vi "Dashboard Main.vi"() -> ()   [LabVIEW 2014]
uses:
  Typedefs/StackerStates.ctl
  Typedefs/Arm States.ctl
  Typedefs/ClawStates.ctl
  <vilib>/event_ctls.llb/eventvkey.ctl
  <vilib>/Rock Robotics/WPI/Dashboard/WPI_DashboardLogging Global.vi
  <vilib>/Rock Robotics/Network Tables/SD Read Boolean.vi
  <vilib>/Rock Robotics/Network Tables/SD Read Number.vi
  <vilib>/Rock Robotics/Network Tables/SD Read String Array.vi
  <vilib>/Utility/config.llb/Write Key (String).vi
  <vilib>/Utility/config.llb/Write Key (I32).vi
  <vilib>/Utility/config.llb/NI_LVConfig.lvlib
panel:
  in  "TCP":refnum<k5>
  in  "Rec Mode":enum32{"Stop", "Record", "Playback"}(radio)
  in  "Vision":u16(ring) items=["Camera Off", "USB Camera SW", "USB Camera HW", "IP Camera"]
  out "Camera IP":string
  out "Image Message":string="Timeout in Camera Communications"
  in  "Dashboard Tab":T1(tab)
  in  "Camera Settings":T2={"Frame Rate"=30, "Compression"=30, "Size"=1} {"Frame Rate" scale=1.0..30.0; "Size" items=["640x480", "320x240", "160x120"]}
  out "MotorChart R":cluster{"Numeric":dbl, "Numeric":dbl}(graph)
  out "MotorChart L":T3(graph)
  out "MotorSliders R":cluster{"MotorSlide1":dbl, "MotorSlide2":dbl} {"MotorSlide2" scale=-1.0..1.0 scale format="%#_2e"; "MotorSlide1" scale=-1.0..1.0 scale format="%#_2e"}
  out "MotorSliders L":T4 {"MotorSlide4 2" scale=0.0..14.0 scale format="%#_2e"; "MotorSlide2" scale=-1.0..1.0 scale format="%#_2e"; "MotorSlide1" scale=-1.0..1.0 scale format="%#_2e"}
  out "Gyro":dbl(knob) scale=0.0..360.0
  out "JS1 Z":dbl(slide) scale=-1.0..1.0 scale format="%#_2e"
  out "JS1 Graph":cluster{"X":dbl, "Y":dbl}[](graph)
  out "JS1 Buttons":T5
  out "JS2 Z":dbl(slide) scale=-1.0..1.0 scale format="%#_2e"
  out "JS2 Graph":cluster{"X":dbl, "Y":dbl}[](graph)
  out "JS2 Buttons":T5
  out "Mode":T6(ring)=enum."Auto Disabled"
  in  "DB Camera Config":bool
  out "fps":dbl format="%#.1g"
  out "Mbps":dbl format="%#.1g"
  out "Mbps 2":bool
  in  "DB/String 9":string
  in  "DB/String 8":string
  in  "DB/String 7":string
  in  "DB/String 6":string
  in  "DB/String 5":string
  in  "DB/String 4":string
  in  "DB/String 3":string
  in  "DB/String 2":string
  in  "DB/String 1":string
  in  "DB/String 0":string
  in  "DB/Slider 0":dbl(slide) scale=0.0..5.0
  in  "DB/Slider 1":dbl(slide) scale=0.0..5.0
  in  "DB/Slider 2":dbl(slide) scale=0.0..5.0
  in  "DB/Slider 3":dbl(slide) scale=0.0..5.0
  out "DB/LED 3":bool
  out "DB/LED 2":bool
  out "DB/LED 1":bool
  out "DB/LED 0":bool
  in  "DB/Button 3":bool
  in  "DB/Button 2":bool
  in  "DB/Button 1":bool
  in  "DB/Button 0":bool caption="New Name"
  out "Claw On":bool
  out "Intake On":bool
  out "Right Throttle":dbl
  out "Comp Bot":bool
  out "Intake Sensor Enabled":bool
  out "Number of Totes":u8
  out "Compressor On":bool
  out "Intake Sees Tote":bool
  out "Stacker Sees Tote":bool
  out "Tusks Up":bool
  out "Stacker On":bool
  out "Compressor Enabled":bool
  out "Stacker State to Index":T7
  out "Arm State":T8
  out "Claw State":T9
  out "Auto Mode":string
  out "Left Throttle":dbl
  out "Claw Sees Can":bool
  out "Stack Clamp Locked?":bool
  in  "Test Slider":dbl(slide) scale=0.0..100.0 scale format="%#_3g"
  in  "On/Off":bool caption="Solenoid"
  in  "Test Name":u16(ring) items=["Select the test to run...", "Example Test", "-------------------------------", "List of tests is built in robot code.", "Replace with your own automated tests."]
  in  "Test Tree":string(tree)
  in  "Motor":cluster{"Value":dbl, "Enable":bool} {"Value" scale=-1.0..1.0 scale format="%#_3g"}
  out "Progress":T10 {"Test Progress" scale=0.0..100.0}
  in  "Rev/Fwd":cluster{"Forward":bool, "Reverse":bool}
  in  "Test Ring":u16(ring) items=["Monochrome", "Color"]
  in  "Listbox":i32(listbox)
  out "Tree":string(tree)
  out "Camera Image":T11(plugin-control)
  out "Boolean":bool
  # "Left"
  # "Front"
  # "Right"
  # "Battery"
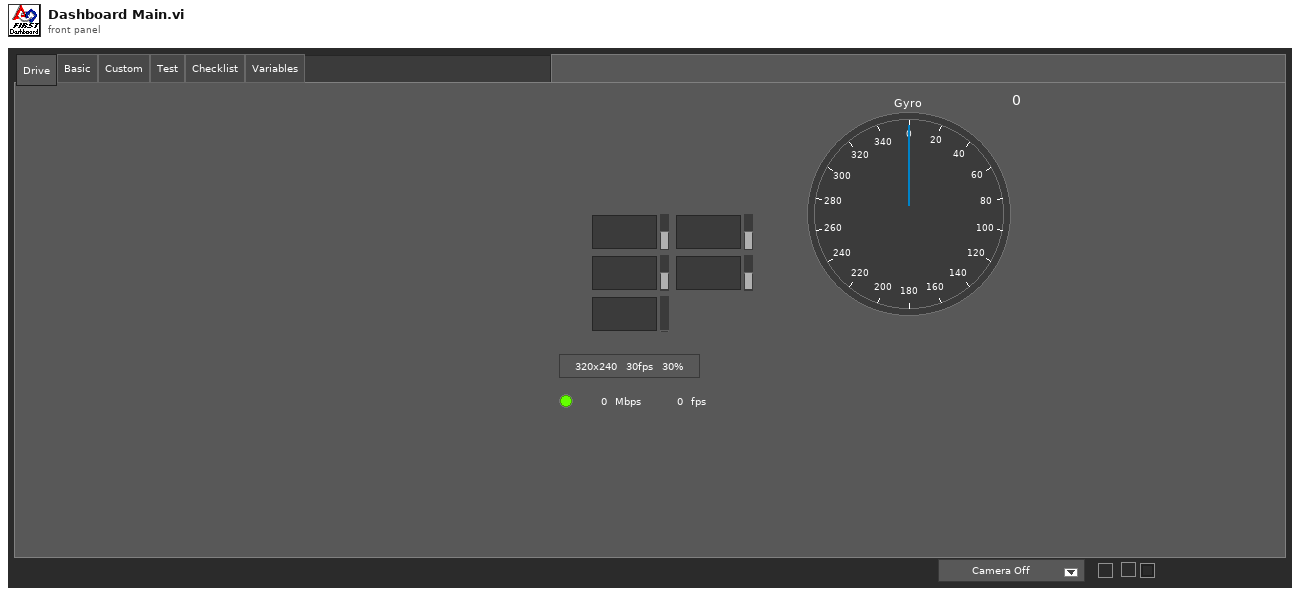
[diagram p1: front panel]
types:
  T1 = enum32{"Drive", "Basic", "Custom", "Test", "Checklist", "Variables"}
  T2 = cluster{"Frame Rate":i32, "Compression":i32, "Size":u16}
  T3 = cluster{"Numeric":dbl, "Numeric":dbl, "Battery V":dbl}
  T4 = cluster{"MotorSlide1":dbl, "MotorSlide2":dbl, "MotorSlide4 2":dbl}
  T5 = cluster{bool, bool, bool, bool, bool, bool, bool, bool, bool, bool, bool, bool}
  T6 = enum8{"Tele-Op Disabled", "Tele-Op Enabled", "Auto Disabled", "Auto Enabled", "Test Disabled", "Test Enabled", "Disconnected", "No Code", "E-Stop"}
  T7 = typedef "StackerStates.ctl" = enum16{"Manual ", "Hold", "Hold5", "Hold6", "GetTote", "DropStack", "Hover", "Hover5", "Wait for Up", "DecideHold", "DownTimerPeriod", "Prep Intake for Drop", "Check Arm before 5", "Make Arm ready for 5", "Check Arm before 6", "Make Arm ready for 6", "Delay for 5", "Delay for 6"}
  T8 = typedef "Arm States.ctl" = enum16{"Arm Manual ", "Ground", "Step", "1 Tote", "2 Tote", "3 Tote", "4 Tote", "5 Tote", "6 Tote", "Flip Can Arm", "Grab Can in auto"}
  T9 = typedef "ClawStates.ctl" = enum16{"Claw Manual ", "Claw Open", "Claw Closed", "Claw Slight Open", "Flip Can"}
  T10 = cluster{"Test Progress":u8, "Test Progress Text":string}
  T11 = typedef "IMAQ Image.ctl" = refnum<image>
  T12 = typedef "Image Type" = u32
  T13 = cluster{"Camera Image":refnum<vi>, "Dashboard Tab":refnum<vi>, "Boolean":refnum<vi>, "Vision":refnum<vi>, "Rec Mode":refnum<vi>, "Test Slider":refnum<vi>, "On/Off ":refnum<vi>, "Test Ring":refnum<vi>, "Rev/Fwd":refnum<vi>, "Test Name":refnum<vi>, "Motor":refnum<vi>, "Progress":refnum<vi>, "CheckList":refnum<vi>, "Tree":refnum<vi>, "Test Tree":refnum<vi>}
  T14 = cluster{"Error Strings":string, "Disable Counts":cluster{u16, u16}, "Rail Faults":cluster{u16, u16, u16}, "Robot IP":string, "DB Mode":u8, "Event Info":cluster{"Name":string, "Type":u8, "Number":u16, "Replay":u8}, "Camera Addr":string}
  T15 = cluster{"Storage":cluster{"Disk Free":u64, "RAM Block":u32, "RAM free":u32}, "CPU Utilization":cluster{"CPU % ISR":sgl, "CPU % Time Crit":sgl, "CPU % Timed Str":sgl, "CPU % High":sgl, "CPU % Above":sgl, "CPU % Normal":sgl, "CPU % Low":sgl}, "CAN":cluster{"% Bus Utilization":sgl, "Bus Off Cnt":u32, "TX_FIFO Full Cnt":u32, "Receive Error Cnt":u8, "Transmit Error Cnt":u8}, "HID":cluster{"HID Outputs":u32, "Rumble Low":u16, "Rumble High":u16}[]}
  T16 = cluster{"Status bits":cluster{"Test Mode":bool, "Autonomous":bool, "Enabled":bool, "Code Start":bool, "Brownout":bool, "Reserved 2":bool, "Reserved 3":bool, "E-Stop":bool}, "Code Trace":cluster{"Disabled":bool, "TeleOp":bool, "Auto":bool, "Test":bool}, "Controller Type":enum16{"unknown", "cRIO", "roboRio"}, "Code?":enum16{"unknown", "noCode", "code"}, "Battery V":dbl}
  T17 = cluster{"Control Bits":cluster{"TestMode":bool, "Autonomous":bool, "Enabled":bool, "FMS Present":bool, bool, bool, bool, "E-Stop":bool}, "Team Station ":u8, "Countdown":sgl, "Joystick Values":cluster{"Axes":dbl[], "Buttons":bool[], "POVs":i16[]}[]}
  T18 = cluster{"Axes":dbl[], "Buttons":bool[], "POVs":i16[]}[]
  T19 = cluster{"Axes":dbl[], "Buttons":bool[], "POVs":i16[]}
  T20 = cluster{"Buttons[0]":bool, "Buttons[1]":bool, "Buttons[2]":bool, "Buttons[3]":bool, "Buttons[4]":bool, "Buttons[5]":bool, "Buttons[6]":bool, "Buttons[7]":bool, "Buttons[8]":bool, "Buttons[9]":bool, "Buttons[10]":bool, "Buttons[11]":bool}
  T21 = typedef "NI_LVConfig.lvlib/Config Data RefNum.ctl" = refnum<k1>
  T22 = cluster{"Operation":enum16{"Update", "Clear"}, "Color Box":u32}[]
  T23 = typedef "eventvkey.ctl" = enum16{"ASCII", "Enter", "Return", "Shift", "Ctrl", "Alt", "Cmd", "Opt", "Caps", "NumLock", "Clear", "Break", "Up", "Down", "Left", "Right", "Insert", "Delete", "Home", "End", "PageUp", "PageDown", "Escape", "Help", "Pause", "ScrollLock", "F1", "F2", "F3", "F4", "F5", "F6", "F7", "F8", "F9", "F10", "F11", "F12", "F13", "F14", "F15", "F16", "F17", "F18", "F19", "F20", "F21", "F22", "F23", "F24", "Play", "VolumeUp", "VolumeDown", "Mute", "Two Byte Char"}
  T24 = cluster{"Image Size":bool, "Image Type":bool, "Pixel Value":bool, "ROI Information":bool, "Zoom Factor":bool}
  T25 = enum8{"Enabled", "Disabled", "Disabled and Grayed Out"}
  T26 = cluster{"Operation":enum16{"Update", "Clear"}, "Color Box":u32}
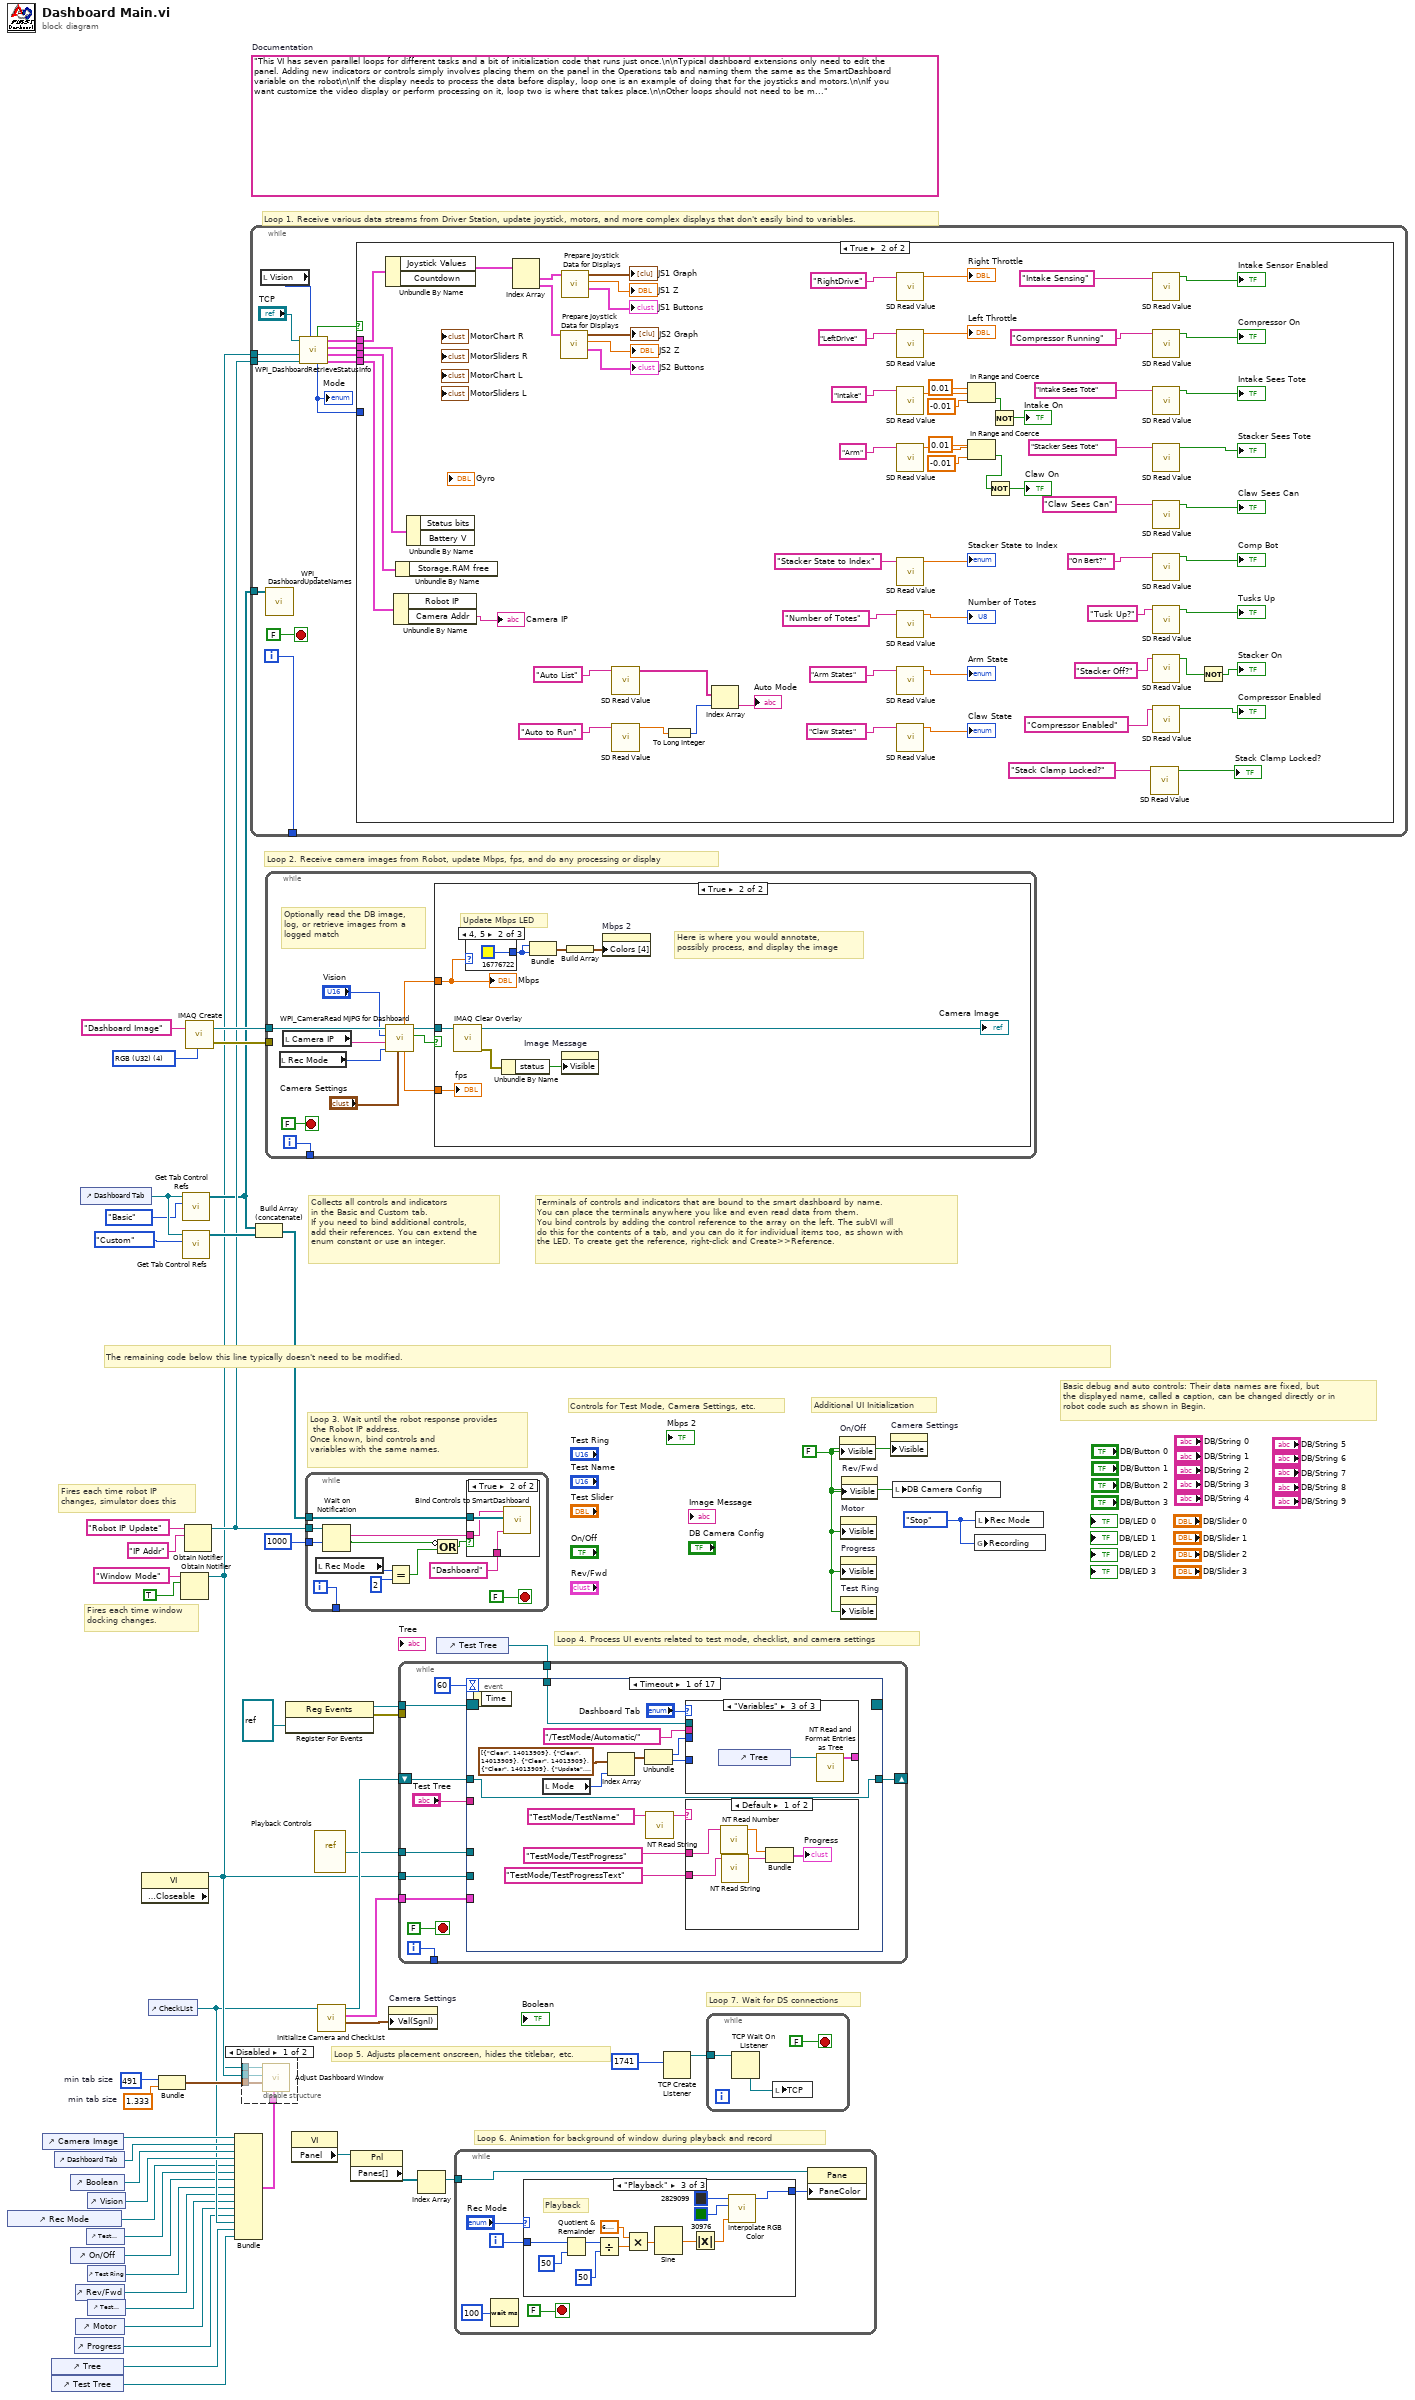
[diagram p0: block diagram]
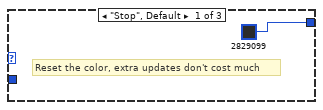
[diagram p4: hidden frame]
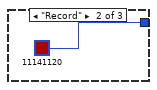
[diagram p5: hidden frame]
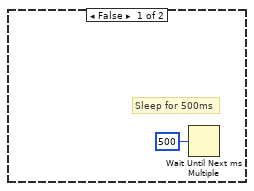
[diagram p7: hidden frame]
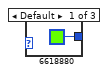
[diagram p8: hidden frame]
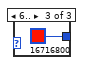
[diagram p9: hidden frame]
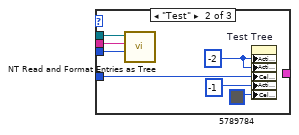
[diagram p11: hidden frame]
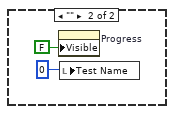
[diagram p12: hidden frame]
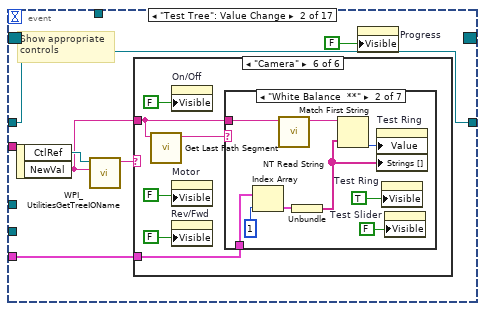
[diagram p13: hidden frame]
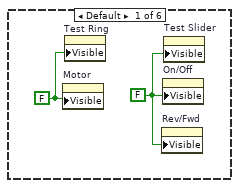
[diagram p14: hidden frame]
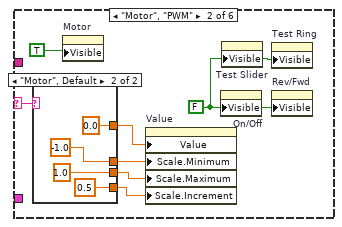
[diagram p15: hidden frame]
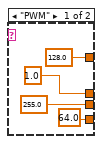
[diagram p16: hidden frame]
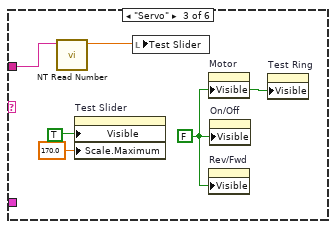
[diagram p17: hidden frame]
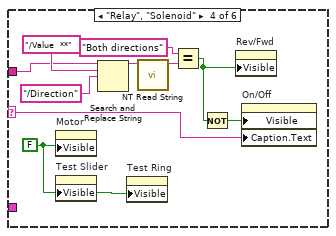
[diagram p18: hidden frame]
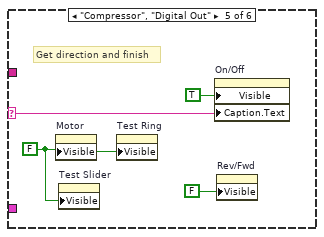
[diagram p19: hidden frame]
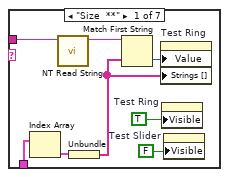
[diagram p20: hidden frame]
diagram:
  w24 = 491  # min tab size
  w23 = 1.333  # min tab size
  w32 = enum32{"Stop", "Record", "Playback"}."Stop" ("Rec Mode")
  w6 = FALSE ("Visible")
  (unwired) "This VI has seven parallel loops for different tasks and a bit of initialization code that runs just once.\n\nTypical dashboard extensions only need to edit the panel. Adding new indicators or controls simply involves placing them on the panel in the Operations tab and naming them the same as the SmartDashboard variable on the robot\n\nIf the display needs to process the data before display, loop one is an example of doing that for the joysticks and motors.\n\nIf you want customize the video display or perform processing on it, loop two is where that takes place.\n\nOther loops should not need to be modified. They are pretty standard, and document the task they perform."  # Documentation
  w52 = T12 4 items=["Grayscale (U8)", "Grayscale (I16)", "Grayscale (SGL)", "Complex (CSG)", "RGB (U32)", "HSL (U32)", "RGB (U64)"] ("Image Type")
  # "Loop 7. Wait for DS connections"
  # "Basic debug and auto controls: Their data names are fixed, but\nthe displayed name, called a caption, can be changed directly or in\nrobot code such as shown in Begin."
  # "Controls for Test Mode, Camera Settings, etc."
  # "Additional UI Initialization"
  # "Loop 6. Animation for background of window during playback and record"
  # "Fires each time robot IP\nchanges, simulator does this"
  # "Fires each time window\ndocking changes."
  # "Collects all controls and indicators\nin the Basic and Custom tab.\nIf you need to bind additional controls,\nadd their references. You can extend the\nenum constant or use an integer."
  # "The remaining code below this line typically doesn't need to be modified."
  # "Loop 4. Process UI events related to test mode, checklist, and camera settings"
  # "Terminals of controls and indicators that are bound to the smart dashboard by name.\nYou can place the terminals anywhere you like and even read data from them.\nYou bind controls by adding the control reference to the array on the left. The subVI will\ndo this for the contents of a tab, and you can do it for individual items too, as shown with\nthe LED. To create get the reference, right-click and Create>>Reference."
  # "Loop 3. Wait until the robot response provides\n the Robot IP address.\nOnce known, bind controls and\nvariables with the same names."
  # "Loop 5. Adjusts placement onscreen, hides the titlebar, etc."
  # "Loop 1. Receive various data streams from Driver Station, update joystick, motors, and more complex displays that don't easily bind to variables."
  # "Loop 2. Receive camera images from Robot, update Mbps, fps, and do any processing or display"
  n1 = control-ref of="Rec Mode"() -> (w12:refnum<vi>)
  n2 = control-ref of="Camera Image"() -> (w27:refnum<vi>)
  n3 = control-ref of="Tree"() -> (w16:refnum<vi>)
  n4 = control-ref of="Test Tree"() -> (w15:refnum<vi>)
  n5 = control-ref of="Dashboard Tab"() -> (w26:refnum<vi>)
  n6 = control-ref of="Boolean"() -> (w21:refnum<vi>)
  n7 = control-ref of="On/Off"() -> (w10:refnum<vi>)
  n8 = control-ref of="Progress"() -> (w7:refnum<vi>)
  n9 = control-ref of="Rev/Fwd"() -> (w8:refnum<vi>)
  n10 = control-ref of="Motor"() -> (w13:refnum<vi>)
  n11 = control-ref of="Dashboard Tab"() -> (w30:refnum<vi>)
  n12 = control-ref of="Test Slider"() -> (w11:refnum<vi>)
  n13 = control-ref of="Vision"() -> (w25:refnum<vi>)
  n14 = control-ref of="Test Ring"() -> (w9:refnum<vi>)
  n15 = control-ref of="Test Name"() -> (w14:refnum<vi>)
  n16 = property class="VI" props=["Front Panel.Closeable"]() -> (reference out=w31:refnum<vi>)  [unwired: 2 in, 2 out]
  n17 = control-ref of="CheckList"() -> (w17:refnum<vi>)
  n18 = Bundle("min tab size"=w24, "min tab size"=w23) -> (w22:cluster{"min tab size":i32, "min tab size":dbl})  [unwired: 1 in]
  n19 = Obtain Notifier(name (unnamed)="Window Mode", notification data type=TRUE) -> (notifier out=w3:refnum<notifier>)  [unwired: 2 in, 2 out]
  n20 = call <vilib>:"Get Tab Control Refs.vi"("Page Index"=T1."Basic" ("Dashboard Tab"), "TabControl in"=w30) -> ("ControlsOnPage"=w4:refnum<vi>[])  [unwired: 9 in]
  n21 = call <vilib>:"Get Tab Control Refs.vi"("Page Index"=T1."Custom" ("Dashboard Tab"), "TabControl in"=w30) -> ("ControlsOnPage"=w29:refnum<vi>[])  [unwired: 9 in]
  n22 = Obtain Notifier(name (unnamed)="Robot IP Update", notification data type="IP Addr" ("name (unnamed)")) -> (notifier out=w5:refnum<notifier>)  [unwired: 2 in, 2 out]
  n23 = call "IMAQ Create"("Image Name"="Dashboard Image", "Image Type"=w52) -> ("New Image"=w50:T11, "error out"=w49:errorcluster)  [unwired: 2 in, 1 out]
  n24 = Bundle("Camera Image"=w27, "Dashboard Tab"=w26, "Boolean"=w21, "Vision"=w25, "Rec Mode"=w12, "Test Slider"=w11, "On/Off"=w10, "Test Ring"=w9, "Rev/Fwd"=w8, "Test Name"=w14, "Motor"=w13, "Progress"=w7, "CheckList"=w17, "Tree"=w16, "Test Tree"=w15) -> (w18:T13)  [unwired: 1 in]
  n25 = disable-structure shown="Disabled" {
    disable-tunnel: w31 -> [w56 _]
    disable-tunnel: w22 -> [w55 _]
    disable-tunnel: w18 -> [w54 _]
    disable-tunnel: w3 -> [w53 _]
    frame Disabled {
      n26 = call "Adjust Dashboard Window.vi"("Sizing Refnums"=w54, "Size Constraints"=w55, "VI"=w56, "Notifier in"=w53) -> ()  [unwired: 8 in]
    }
    frame Enabled {
    }
  }
  n27 = while {
    tunnel: [w68] -> _
    tunnel: w5 -> [w62]
    tunnel: w4 -> [w61]
    tunnel: w3 -> [w57]
    i -> [w68]
    stop <- FALSE stop-if-true
    n28 = local read "Vision"() -> (w59:u16)
    n29 = call <vilib>:"WPI_DashboardUpdateNames.vi"("Controls on Tab"=w61) -> ()  [unwired: 11 in]
    n30 = call <vilib>:"WPI_DashboardRetrieveStatusInfo.vi"("Vision"=w59, "Binding Refnum"=w62, "Window Mode Notifier"=w57, "TCP Cnx"="TCP") -> ("Power and Errors"=w63:T14, "Robot Metrics"=w66:T15, "Status Info"=w67:T16, "Control Info"=w64:T17, "Robot Mode"=w60:T6, "Process?"=w65:bool)  [unwired: 2 in]
    "Mode" <- w60
    n31 = case shown="True" w65 {
      tunnel: w67 -> [_ w134]
      tunnel: w66 -> [_ w133]
      tunnel: w64 -> [_ w132]
      tunnel: w63 -> [_ w131]
      tunnel: w60 -> [_ _]
      frame False {
      }
      frame True {
        n32 = Unbundle By Name(w132) -> ("Joystick Values"=w130:T18)  [unwired: 1 out]
        n33 = Unbundle By Name(w131) -> ("Camera Addr"=→"Camera IP":string)  [unwired: 1 out]
        n34 = Unbundle By Name(w133) -> ()  [unwired: 1 out]
        n35 = Unbundle By Name(w134) -> ()  [unwired: 2 out]
        n36 = Index Array(array=w130) -> (element #1=w129:T19, element #2=w124:T19)  [unwired: 2 in]
        n37 = call "Prepare Joystick Data for Displays.vi"("Joystick Values"=w124) -> ("Buttons"=→"JS2 Buttons":T20, "Z Axis"=→"JS2 Z":dbl, "Cartesian Data"=→"JS2 Graph":cluster{"X axis":dbl, "X axis":dbl}[])  [unwired: 8 in]
        n38 = call "Prepare Joystick Data for Displays.vi"("Joystick Values"=w129) -> ("Buttons"=→"JS1 Buttons":T20, "Z Axis"=→"JS1 Z":dbl, "Cartesian Data"=→"JS1 Graph":cluster{"X axis":dbl, "X axis":dbl}[])  [unwired: 8 in]
        n39 = call-poly <vilib>:"SD Read Value.vi"("Name"="Auto List") -> ("String Array"=w89:string[])  [unwired: 9 in, 1 out]
        n40 = call-poly <vilib>:"SD Read Value.vi"("Name"="Auto to Run") -> ("Numeric"=w88:dbl)  [unwired: 8 in, 2 out]
        n41 = To Long Integer(number=w88) -> (32bit integer=w87:i32)
        n42 = Index Array(array=w89, index=w87) -> (element=→"Auto Mode":string)
        n43 = call-poly <vilib>:"SD Read Value.vi"("Name"="RightDrive") -> ("Numeric"=→"Right Throttle":dbl)  [unwired: 8 in, 2 out]
        n44 = call-poly <vilib>:"SD Read Value.vi"("Name"="LeftDrive") -> ("Numeric"=→"Left Throttle":dbl)  [unwired: 8 in, 2 out]
        n45 = call-poly <vilib>:"SD Read Value.vi"("Name"="Intake") -> ("Numeric"=w83:dbl)  [unwired: 8 in, 2 out]
        n46 = call-poly <vilib>:"SD Read Value.vi"("Name"="Arm") -> ("Numeric"=w78:dbl)  [unwired: 8 in, 2 out]
        n47 = call-poly <vilib>:"SD Read Value.vi"("Name"="Stacker State to Index") -> ("Numeric"=→"Stacker State to Index":dbl)  [unwired: 8 in, 2 out]
        n48 = call-poly <vilib>:"SD Read Value.vi"("Name"="Number of Totes") -> ("Numeric"=→"Number of Totes":dbl)  [unwired: 8 in, 2 out]
        n49 = call-poly <vilib>:"SD Read Value.vi"("Name"="Arm States") -> ("Numeric"=→"Arm State":dbl)  [unwired: 8 in, 2 out]
        n50 = call-poly <vilib>:"SD Read Value.vi"("Name"="Claw States") -> ("Numeric"=→"Claw State":dbl)  [unwired: 8 in, 2 out]
        n51 = In Range and Coerce(upper limit=0.01, x=w83, lower limit=-0.01 ("upper limit")) -> (In Range?=w76:bool)  [unwired: 1 out]
        n52 = In Range and Coerce(upper limit=0.01, x=w78, lower limit=-0.01 ("upper limit")) -> (In Range?=w74:bool)  [unwired: 1 out]
        n53 = Not(x=w74) -> (.not. x?=→"Claw On":bool)
        n54 = Not(x=w76) -> (.not. x?=→"Intake On":bool)
        n55 = call-poly <vilib>:"SD Read Value.vi"("Name"="Stack Clamp Locked?") -> ("Boolean"=→"Stack Clamp Locked?":bool)  [unwired: 8 in, 2 out]
        n56 = call-poly <vilib>:"SD Read Value.vi"("Name"="Intake Sensing") -> ("Boolean"=→"Intake Sensor Enabled":bool)  [unwired: 8 in, 2 out]
        n57 = call-poly <vilib>:"SD Read Value.vi"("Name"="Compressor Running") -> ("Boolean"=→"Compressor On":bool)  [unwired: 8 in, 2 out]
        n58 = call-poly <vilib>:"SD Read Value.vi"("Name"="Intake Sees Tote") -> ("Boolean"=→"Intake Sees Tote":bool)  [unwired: 8 in, 2 out]
        n59 = call-poly <vilib>:"SD Read Value.vi"("Name"="Stacker Sees Tote") -> ("Boolean"=→"Stacker Sees Tote":bool)  [unwired: 8 in, 2 out]
        n60 = call-poly <vilib>:"SD Read Value.vi"("Name"="Claw Sees Can") -> ("Boolean"=→"Claw Sees Can":bool)  [unwired: 8 in, 2 out]
        n61 = call-poly <vilib>:"SD Read Value.vi"("Name"="On Bert?") -> ("Boolean"=→"Comp Bot":bool)  [unwired: 8 in, 2 out]
        n62 = call-poly <vilib>:"SD Read Value.vi"("Name"="Tusk Up?") -> ("Boolean"=→"Tusks Up":bool)  [unwired: 8 in, 2 out]
        n63 = call-poly <vilib>:"SD Read Value.vi"("Name"="Stacker Off?") -> ("Boolean"=w72:bool)  [unwired: 8 in, 2 out]
        n64 = call-poly <vilib>:"SD Read Value.vi"("Name"="Compressor Enabled") -> ("Boolean"=→"Compressor Enabled":bool)  [unwired: 8 in, 2 out]
        n65 = Not(x=w72) -> (.not. x?=→"Stacker On":bool)
      }
    }
  }
  n66 = Build Array (concatenate)(w4, w29) -> (w28:refnum<vi>[])
  n67 = while {
    tunnel: w50 -> [w143]
    tunnel: w49 -> [_]
    tunnel: [w144] -> _
    i -> [w144]
    stop <- FALSE stop-if-true
    # "Optionally read the DB image,\nlog, or retrieve images from a\nlogged match"
    n68 = local read "Rec Mode"() -> (w137:enum32{"Stop", "Record", "Playback"})
    n69 = local read "Camera IP"() -> (w135:string)
    n70 = call <vilib>:"WPI_CameraRead MJPG for Dashboard.vi"("Camera Settings"="Camera Settings", "Rec Mode"=w137, "Camera IP"=w135, "Camera Mode"="Vision", "Refnum in"=w143) -> ("Active"=w141:bool, "Refnum out"=w142:T11, "FPS"=w140:dbl, "Bandwidth (Mbps)"=w139:dbl)  [unwired: 3 in]
    n71 = case shown="True" w141 {
      tunnel: w142 -> [_ w150]
      tunnel: w139 -> [_ w149]
      tunnel: w140 -> [_ w147]
      frame False {
        # "Sleep for 500ms"
        n72 = Wait Until Next ms Multiple(millisecond multiple=u32 500) -> ()  [unwired: 1 out]
      }
      frame True {
        # "Here is where you would annotate,\npossibly process, and display the image"
        # "Update Mbps LED"
        n73 = call "IMAQ Clear Overlay"("Image"=w150) -> ("error out"=w154:errorcluster, "Image Out"=→"Camera Image":T11)  [unwired: 2 in, 7 out]
        n74 = case shown="4, 5" w149 {
          tunnel: [u32 6618880 ("Color Box") u32 16776722 ("Color Box") u32 16716800 ("Color Box")] -> w151
          frame Default {
          }
          frame 4, 5 {
          }
          frame 6.. {
          }
        }
        n75 = Unbundle By Name(w154) -> ("status"=w155:bool)
        n76 = Bundle("Color Box"=w151, "Color Box"=w151) -> (w153:cluster{"Color Box":u32, "Color Box":u32})  [unwired: 1 out]
        n77 = property on="Image Message" class="Str"("Visible"=w155) -> ()  [unwired: 2 in, 2 out]
        n78 = Build Array(w153) -> (w152:cluster{"Color Box":u32, "Color Box":u32}[])
        n79 = property on="Mbps 2" class="Bool (strict)"("Colors [4]"=w152) -> ()  [unwired: 2 in, 2 out]
        "Mbps" <- w149
        "fps" <- w147
      }
    }
  }
  n80 = register-events(refnum<vi> refnum) -> (reference out=w36:refnum<event-registration>, error out=w35:errorcluster)  [unwired: 2 in]
  n81 = property class="VI"() -> ("Panel"=w39:refnum<vi>)  [unwired: 2 in, 2 out]
  n82 = while {
    tunnel: w28 -> [w170]
    tunnel: w5 -> [w168]
    tunnel: [w166] -> _
    tunnel: u32 1000 ("milliseconds to wait") -> [w165]
    i -> [w166]
    stop <- FALSE stop-if-true
    n83 = local read "Rec Mode"() -> (w161:enum32{"Stop", "Record", "Playback"})
    n84 = Wait on Notification(notifier=w168, timeout in ms (-1)=w165) -> (notification=w167:string, timed out?=w163:bool)  [unwired: 2 in, 2 out]
    n85 = Equal?(x=w161, y=u16 2 ("Rec Mode")) -> (x = y?=w162:bool)
    n86 = Compound Arithmetic op=OR(invert w163, w162) -> (w164:bool)
    n87 = case shown="True" w164 {
      tunnel: w170 -> [_ w173]
      tunnel: w167 -> [_ w172]
      tunnel: "Dashboard" -> [_ w171]
      frame False {
      }
      frame True {
        n88 = call <vilib>:"Bind Controls to SmartDashboard.vi"("Client Name"=w171, "Bound Control Refs"=w173, "Server IP Address"=w172) -> ()  [unwired: 9 in]
      }
    }
  }
  n89 = vi-ref "Playback Controls.vi"() -> (w37:refnum<vi>)
  n90 = call "Initialize Camera and CheckList.vi"("ListBox in"=w17) -> ("Cluster"=w43:cluster{"value":i32, "value":i32, "index":i32}, "Array"=w44:cluster{string[]}[], "File Refnum"=w42:T21)  [unwired: 8 in]
  n91 = property class="Pnl"(reference=w39) -> ("Panes[]"=w40:refnum<vi>[])  [unwired: 1 in, 2 out]
  n92 = property on="Camera Settings" class="Clust (strict)"("Val(Sgnl)"=w43) -> ()  [unwired: 2 in, 2 out]
  n93 = Index Array(array=w40) -> (element=w38:refnum<vi>)  [unwired: 1 in]
  n94 = control-ref of="Test Tree"() -> (w41:refnum<vi>)
  n95 = while {
    tunnel: w44 -> [w181]
    shift-right: [w180] -> _
    shift-left: w42 -> [w179]
    tunnel: [w178] -> _
    tunnel: w41 -> [w177]
    tunnel: w37 -> [w176]
    tunnel: w36 -> [w175]
    tunnel: w35 -> [_]
    tunnel: w31 -> [w174]
    i -> [w178]
    stop <- FALSE stop-if-true
    n96 = event shown="[0] Timeout" {
      selector: w175 -> [_ _ _ _ _ _ _ _ _ _ _ _ _ _ _ _ _]
      dyn-events: [_ _ _ _ _ _ _ _ _ _ _ _ _ w419 _ _ _] -> _
      timeout: u32 60 ("milliseconds to wait") -> [_ _ _ _ _ _ _ _ _ _ _ _ _ _ _ _ _]
      tunnel: w177 -> [w193 _ _ _ _ _ _ _ _ _ _ _ _ _ _ _ _]
      tunnel: "Test Tree" -> [_ _ _ _ _ _ _ _ w388 w396 w398 w402 w410 _ _ _ _]
      tunnel: w181 -> [_ w215 _ _ _ _ w352 w382 _ _ _ _ _ _ _ _ _]
      tunnel: [w189 w214 w313 w318 w326 w338 w351 w375 w387 w394 w397 w401 w409 w421 w435 w436 w446] -> w180
      tunnel: w179 -> [w189 w214 w313 w318 w326 w338 w350 w375 w387 w394 w397 w401 w409 w421 w435 w436 w446]
      tunnel: w176 -> [_ _ _ _ _ _ _ _ _ _ _ _ _ w422 _ w439 _]
      tunnel: w174 -> [_ _ _ _ _ _ _ _ _ _ _ _ _ w417 _ _ _]
      event Timeout {
        n97 = event-data() -> ()  [unwired: 1 in, 1 out]
        n98 = local read "Mode"() -> (w192:T6)
        n99 = Index Array(array=T22 [{"Operation"=enum."Clear", "Color Box"=14013909}, {"Operation"=enum."Clear", "Color Box"=14013909}, {"Operation"=enum."Clear", "Color Box"=14013909}, {"Operation"=enum."Clear", "Color Box"=14013909}, {"Operation"=enum."Update", "Color Box"=14013909}, {"Operation"=enum."Update", "Color Box"=16777215}, {"Operation"=enum."Clear", "Color Box"=14013909}, {"Operation"=enum."Clear", "Color Box"=14013909}, {"Operation"=enum."Clear", "Color Box"=14013909}], index=w192) -> (element=w187:T26)
        n100 = Unbundle(w187) -> ("Operation"=w186:enum16{"Update", "Clear"}, "Color Box"=w185:u32)
        n101 = call <vilib>:"NT Read String.vi"("Name"="TestMode/TestName") -> ("String"=w196:string)  [unwired: 9 in, 1 out]
        n102 = case shown="\"Variables\"" "Dashboard Tab" {
          tunnel: w193 -> [_ w204 _]
          tunnel: "/TestMode/Automatic/" ("Name Pattern") -> [_ w203 _]
          tunnel: w186 -> [_ w202 _]
          tunnel: [_ _ w206] -> _
          tunnel: w185 -> [_ w198 _]
          frame "Custom", Default {
          }
          frame "Test" {
            w201 = -2 ("Active Item:Row Number")
            n103 = call <vilib>:"NT Read and Format Entries as Tree.vi"("Operation"=w202, "Name Pattern"=w203, "Tree Refnum"=w204) -> ()  [unwired: 7 in, 2 out]
            n104 = property on="Test Tree" class="Tree (strict)"("Active Item Row Number"=w201, "ActiveColNum"=w201, "CellBG"=w198, "Active Item Row Number"=-1 ("Active Item:Row Number"), "CellBG"=u32 5789784 ("Color Box")) -> ()  [unwired: 2 in, 2 out]
          }
          frame "Variables" {
            n105 = control-ref of="Tree"() -> (w205:refnum<vi>)
            n106 = call <vilib>:"NT Read and Format Entries as Tree.vi"("Tree Refnum"=w205) -> ("Formatted Strings"=w206:cluster{"Name":string, "Value":string}[])  [unwired: 9 in, 1 out]
          }
        }
        n107 = case shown="Default" w196 {
          tunnel: "TestMode/TestProgress" ("Name") -> [w208 _]
          tunnel: "TestMode/TestProgressText" ("Name") -> [w207 _]
          frame Default {
            n108 = call <vilib>:"NT Read Number.vi"("Name"=w208) -> ("Numeric"=w209:dbl)  [unwired: 9 in, 1 out]
            n109 = call <vilib>:"NT Read String.vi"("Name"=w207) -> ("String"=w210:string)  [unwired: 9 in, 1 out]
            n110 = Bundle("Numeric"=w209, "String"=w210) -> (→"Progress":cluster{"Numeric":dbl, "String":string})  [unwired: 1 in]
          }
          frame "" {
            n111 = property on="Progress" class="Clust (strict)"("Visible"=FALSE) -> ()  [unwired: 2 in, 2 out]
            n112 = local write "Test Name"(u16 0) -> ()
          }
        }
      }
      event "Test Tree": Value Change {
        # "Show appropriate\ncontrols"
        n113 = event-data() -> ("CtlRef"=w218:refnum<vi>, "NewVal"=w216:string)  [unwired: 1 in]
        n114 = call <vilib>:"WPI_UtilitiesGetTreeIOName.vi"("NewVal"=w216, "TreeControl in"=w218) -> ("I/O Name"=w219:string)  [unwired: 9 in]
        n115 = case shown="\"Camera\"" w219 {
          selector: w219 -> [_ w226 _ w244 w253 _]
          tunnel: w216 -> [_ _ w241 w243 _ w260]
          tunnel: w215 -> [_ _ _ _ _ w259]
          frame Default {
            w221 = FALSE ("Visible")
            w220 = FALSE ("Visible")
            n116 = property on="Motor" class="Clust (strict)"("Visible"=w220) -> ()  [unwired: 2 in, 2 out]
            n117 = property on="Test Ring" class="Ring (strict)"("Visible"=w220) -> ()  [unwired: 2 in, 2 out]
            n118 = property on="Rev/Fwd" class="Clust (strict)"("Visible"=w221) -> ()  [unwired: 2 in, 2 out]
            n119 = property on="On/Off" class="Bool (strict)"("Visible"=w221) -> ()  [unwired: 2 in, 2 out]
            n120 = property on="Test Slider" class="Slide (strict)"("Visible"=w221) -> ()  [unwired: 2 in, 2 out]
          }
          frame "Motor", "PWM" {
            w227 = FALSE ("Visible")
            n121 = case shown="\"Motor\", Default" w226 {
              tunnel: [1.0 ("Value") -1.0 ("Value")] -> w225
              tunnel: [255.0 ("Value") 1.0 ("Value")] -> w224
              tunnel: [128.0 ("Value") 0.0 ("Value")] -> w223
              tunnel: [64.0 ("Value") 0.5 ("Value")] -> w222
              frame "PWM" {
              }
              frame "Motor", Default {
              }
            }
            n122 = property on="Motor" class="Clust (strict)"("Visible"=TRUE) -> ()  [unwired: 2 in, 2 out]
            n123 = property on="Value" class="Slide (strict)"("Value"=w223, "Scale.Minimum"=w225, "Scale.Maximum"=w224, "Scale.Increment"=w222) -> ()  [unwired: 2 in, 2 out]
            n124 = property on="On/Off" class="Bool (strict)"("Visible"=w227) -> ()  [unwired: 2 in, 2 out]
            n125 = property on="Test Slider" class="Slide (strict)"("Visible"=w227) -> ()  [unwired: 2 in, 2 out]
            n126 = property on="Test Ring" class="Ring (strict)"("Visible"=w227) -> ()  [unwired: 2 in, 2 out]
            n127 = property on="Rev/Fwd" class="Clust (strict)"("Visible"=w227) -> ()  [unwired: 2 in, 2 out]
          }
          frame "Servo" {
            w239 = FALSE ("Visible")
            n128 = call <vilib>:"NT Read Number.vi"("Name"=w241) -> ("Numeric"=w240:dbl)  [unwired: 9 in, 1 out]
            n129 = property on="Test Slider" class="Slide (strict)"("Visible"=TRUE, "Scale.Maximum"=170.0 ("Scale.Range:Maximum")) -> ()  [unwired: 2 in, 2 out]
            n130 = local write "Test Slider"(w240) -> ()
            n131 = property on="Motor" class="Clust (strict)"("Visible"=w239) -> ()  [unwired: 2 in, 2 out]
            n132 = property on="Rev/Fwd" class="Clust (strict)"("Visible"=w239) -> ()  [unwired: 2 in, 2 out]
            n133 = property on="On/Off" class="Bool (strict)"("Visible"=w239) -> ()  [unwired: 2 in, 2 out]
            n134 = property on="Test Ring" class="Ring (strict)"("Visible"=w239) -> ()  [unwired: 2 in, 2 out]
          }
          frame "Relay", "Solenoid" {
            w242 = FALSE ("Visible")
            n135 = property on="Motor" class="Clust (strict)"("Visible"=w242) -> ()  [unwired: 2 in, 2 out]
            n136 = property on="Test Slider" class="Slide (strict)"("Visible"=w242) -> ()  [unwired: 2 in, 2 out]
            n137 = Search and Replace String(input string=w243, search string="/Value  **", replace string="/Direction") -> (result string=w249:string)  [unwired: 5 in, 3 out]
            n138 = property on="Test Ring" class="Ring (strict)"("Visible"=w242) -> ()  [unwired: 2 in, 2 out]
            n139 = call <vilib>:"NT Read String.vi"("Name"=w249) -> ("String"=w247:string)  [unwired: 9 in, 1 out]
            n140 = Equal?(x="Both directions", y=w247) -> (x = y?=w245:bool)
            n141 = Not(x=w245) -> (.not. x?=w246:bool)
            n142 = property on="Rev/Fwd" class="Clust (strict)"("Visible"=w245) -> ()  [unwired: 2 in, 2 out]
            n143 = property on="On/Off" class="Bool (strict)"("Visible"=w246, "Caption.Text"=w244) -> ()  [unwired: 2 in, 2 out]
          }
          frame "Compressor", "Digital Out" {
            w252 = FALSE ("Visible")
            # "Get direction and finish"
            n144 = property on="Motor" class="Clust (strict)"("Visible"=w252) -> ()  [unwired: 2 in, 2 out]
            n145 = property on="Test Slider" class="Slide (strict)"("Visible"=w252) -> ()  [unwired: 2 in, 2 out]
            n146 = property on="Test Ring" class="Ring (strict)"("Visible"=w252) -> ()  [unwired: 2 in, 2 out]
            n147 = property on="On/Off" class="Bool (strict)"("Visible"=TRUE, "Caption.Text"=w253) -> ()  [unwired: 2 in, 2 out]
            n148 = property on="Rev/Fwd" class="Clust (strict)"("Visible"=FALSE) -> ()  [unwired: 2 in, 2 out]
          }
          frame "Camera" {
            n149 = call <vilib>:"Get Last Path Segment.vi"("String in"=w260) -> ("String out"=w261:string)  [unwired: 10 in]
            n150 = property on="On/Off" class="Bool (strict)"("Visible"=FALSE) -> ()  [unwired: 2 in, 2 out]
            n151 = property on="Motor" class="Clust (strict)"("Visible"=FALSE) -> ()  [unwired: 2 in, 2 out]
            n152 = property on="Rev/Fwd" class="Clust (strict)"("Visible"=FALSE) -> ()  [unwired: 2 in, 2 out]
            n153 = case shown="\"White Balance  **\"" w261 {
              tunnel: w260 -> [w267 w276 w285 w294 w303 _ w309]
              tunnel: w259 -> [w265 w273 w282 w291 w300 _ _]
              frame "Size  **" {
                n154 = Index Array(array=w265) -> (element=w264:cluster{string[]})  [unwired: 1 in]
                n155 = call <vilib>:"NT Read String.vi"("Name"=w267) -> ("String"=w266:string)  [unwired: 9 in, 1 out]
                n156 = Unbundle(w264) -> (w262:string[])
                n157 = Match First String(2:w262, 3:w266) -> (0:w263:i32)  [unwired: 1 out]
                n158 = property on="Test Ring" class="Ring (strict)"("Value"=w263, "Strings []"=w262) -> ()  [unwired: 2 in, 2 out]
                n159 = property on="Test Ring" class="Ring (strict)"("Visible"=TRUE) -> ()  [unwired: 2 in, 2 out]
                n160 = property on="Test Slider" class="Slide (strict)"("Visible"=FALSE) -> ()  [unwired: 2 in, 2 out]
              }
              frame "White Balance  **" {
                n161 = Index Array(array=w273, index=1) -> (element=w274:cluster{string[]})
                n162 = call <vilib>:"NT Read String.vi"("Name"=w276) -> ("String"=w275:string)  [unwired: 9 in, 1 out]
                n163 = Unbundle(w274) -> (w271:string[])
                n164 = Match First String(2:w271, 3:w275) -> (0:w270:i32)  [unwired: 1 out]
                n165 = property on="Test Ring" class="Ring (strict)"("Value"=w270, "Strings []"=w271) -> ()  [unwired: 2 in, 2 out]
                n166 = property on="Test Ring" class="Ring (strict)"("Visible"=TRUE) -> ()  [unwired: 2 in, 2 out]
                n167 = property on="Test Slider" class="Slide (strict)"("Visible"=FALSE) -> ()  [unwired: 2 in, 2 out]
              }
              frame "Exposure  **" {
                n168 = Index Array(array=w282, index=2) -> (element=w283:cluster{string[]})
                n169 = call <vilib>:"NT Read String.vi"("Name"=w285) -> ("String"=w284:string)  [unwired: 9 in, 1 out]
                n170 = Unbundle(w283) -> (w279:string[])
                n171 = Match First String(2:w279, 3:w284) -> (0:w280:i32)  [unwired: 1 out]
                n172 = property on="Test Ring" class="Ring (strict)"("Value"=w280, "Strings []"=w279) -> ()  [unwired: 2 in, 2 out]
                n173 = property on="Test Ring" class="Ring (strict)"("Visible"=TRUE) -> ()  [unwired: 2 in, 2 out]
                n174 = property on="Test Slider" class="Slide (strict)"("Visible"=FALSE) -> ()  [unwired: 2 in, 2 out]
              }
              frame "Exposure Priority  **" {
                n175 = Index Array(array=w291, index=3) -> (element=w292:cluster{string[]})
                n176 = call <vilib>:"NT Read String.vi"("Name"=w294) -> ("String"=w293:string)  [unwired: 9 in, 1 out]
                n177 = Unbundle(w292) -> (w288:string[])
                n178 = Match First String(2:w288, 3:w293) -> (0:w289:i32)  [unwired: 1 out]
                n179 = property on="Test Ring" class="Ring (strict)"("Value"=w289, "Strings []"=w288) -> ()  [unwired: 2 in, 2 out]
                n180 = property on="Test Ring" class="Ring (strict)"("Visible"=TRUE) -> ()  [unwired: 2 in, 2 out]
                n181 = property on="Test Slider" class="Slide (strict)"("Visible"=FALSE) -> ()  [unwired: 2 in, 2 out]
              }
              frame "Color Enable  **" {
                n182 = Index Array(array=w300, index=4) -> (element=w301:cluster{string[]})
                n183 = call <vilib>:"NT Read String.vi"("Name"=w303) -> ("String"=w302:string)  [unwired: 9 in, 1 out]
                n184 = Unbundle(w301) -> (w297:string[])
                n185 = Match First String(2:w297, 3:w302) -> (0:w298:i32)  [unwired: 1 out]
                n186 = property on="Test Ring" class="Ring (strict)"("Value"=w298, "Strings []"=w297) -> ()  [unwired: 2 in, 2 out]
                n187 = property on="Test Ring" class="Ring (strict)"("Visible"=TRUE) -> ()  [unwired: 2 in, 2 out]
                n188 = property on="Test Slider" class="Slide (strict)"("Visible"=FALSE) -> ()  [unwired: 2 in, 2 out]
              }
              frame Default {
                n189 = property on="Test Ring" class="Ring (strict)"("Visible"=FALSE) -> ()  [unwired: 2 in, 2 out]
                n190 = property on="Test Slider" class="Slide (strict)"("Visible"=FALSE) -> ()  [unwired: 2 in, 2 out]
              }
              frame "Brightness  **", "Color Level  **", "Compression  **", "FPS  **", "Sharpness  **" {
                n191 = call <vilib>:"NT Read Number.vi"("Name"=w309) -> ("Numeric"=w308:dbl)  [unwired: 9 in, 1 out]
                n192 = local write "Test Slider"(w308) -> ()
                n193 = property on="Test Slider" class="Slide (strict)"("Visible"=TRUE, "Scale.Maximum"=100.0 ("Scale.Range:Maximum")) -> ()  [unwired: 2 in, 2 out]
                n194 = property on="Test Ring" class="Ring (strict)"("Visible"=FALSE) -> ()  [unwired: 2 in, 2 out]
              }
            }
          }
        }
        n195 = property on="Progress" class="Clust (strict)"("Visible"=FALSE) -> ()  [unwired: 2 in, 2 out]
      }
      event "Test Name": Mouse Enter {
        # "Populate the ring with the list of tests"
        n196 = event-data() -> ()  [unwired: 1 in, 1 out]
        n197 = call <vilib>:"NT Read String Array.vi"("Name"="TestMode/TestList") -> ("String Array"=w317:string[])  [unwired: 9 in, 1 out]
        n198 = Build Array (concatenate)("Select the test to run...", w317) -> (w316:string[])
        n199 = property on="Test Name" class="Ring (strict)"("Strings []"=w316) -> ()  [unwired: 2 in, 2 out]
      }
      event "Test Name": Value Change {
        w319 = FALSE ("Visible")
        # "Tell the robot the test name to run"
        n200 = event-data() -> ("NewVal"=w323:u16)  [unwired: 1 in]
        n201 = property on="Test Name" class="Ring (strict)"() -> ("Strings []"=w324:string[])  [unwired: 2 in, 2 out]
        n202 = local write "Progress"(T10 {"Test Progress"=0, "Test Progress Text"=""} ("Progress")) -> ()
        n203 = Index Array(array=w324, index=w323) -> (element=w322:string)
        n204 = call <vilib>:"NT Write String.vi"("String"=w322, "Name"="TestMode/TestName") -> ()  [unwired: 9 in, 1 out]
        n205 = property on="Progress" class="Clust (strict)"("Visible"=TRUE) -> ()  [unwired: 2 in, 2 out]
        n206 = property on="Motor" class="Clust (strict)"("Visible"=w319) -> ()  [unwired: 2 in, 2 out]
        n207 = property on="Test Slider" class="Slide (strict)"("Visible"=w319) -> ()  [unwired: 2 in, 2 out]
        n208 = property on="On/Off" class="Bool (strict)"("Visible"=w319) -> ()  [unwired: 2 in, 2 out]
        n209 = property on="Rev/Fwd" class="Clust (strict)"("Visible"=w319) -> ()  [unwired: 2 in, 2 out]
        n210 = property on="Test Ring" class="Ring (strict)"("Visible"=w319) -> ()  [unwired: 2 in, 2 out]
      }
      event "Listbox": Double Click {
        # "Shift clears all"
        # "Update symbols on the listbox"
        n211 = event-data() -> ("PlatMods.Shift"=w327:bool, "Row"=w329:i32)  [unwired: 1 in]
        n212 = case shown="True" w327 {
          tunnel: w329 -> [w333 _]
          tunnel: 1 -> [w332 _]
          frame False {
            n213 = property on="Listbox" class="LstBox (strict)"() -> ("Item Symbols"=w331:i32[])  [unwired: 2 in, 2 out]
            n214 = Replace Array Subset(array=w331, new element=w332, index=w333) -> (w330:i32[])
            n215 = property on="Listbox" class="LstBox (strict)"("Item Symbols"=w330) -> ()  [unwired: 2 in, 2 out]
          }
          frame True {
            w334 = 0 ("Top Row")
            n216 = property on="Listbox" class="LstBox (strict)"() -> ("Number of Rows"=w336:u32)  [unwired: 2 in, 2 out]
            n217 = Initialize Array(0, w336) -> (w335:i32[])
            n218 = property on="Listbox" class="LstBox (strict)"("Top Row"=w334, "Value"=w334, "Item Symbols"=w335) -> ()  [unwired: 2 in, 2 out]
          }
        }
      }
      event "Listbox": Key Down {
        # "Update symbols on the listbox\nLeft and right keys check and uncheck"
        n219 = event-data() -> ("VKey"=w340:T23)  [unwired: 1 in]
        n220 = case shown="\"Left\", \"Right\"" w340 {
          selector: w340 -> [w345 _]
          tunnel: eventvkey."Left" ("VKey") -> [w343 _]
          frame "Left", "Right" {
            n221 = Equal?(x=w343, y=w345) -> (x = y?=w344:bool)
            n222 = Select(t=0, s=w344, f=1) -> (s? t:f=w346:i32)
            n223 = property on="Listbox" class="LstBox (strict)"() -> ("Item Symbols"=w349:i32[])  [unwired: 2 in, 2 out]
            n224 = Replace Array Subset(array=w349, new element=w346, index="Listbox") -> (w348:i32[])
            n225 = property on="Listbox" class="LstBox (strict)"("Item Symbols"=w348) -> ()  [unwired: 2 in, 2 out]
          }
          frame Default {
          }
        }
      }
      event "DB Camera Config": Value Change {
        # "Show or hide the cluster of controls, store in ini file"
        n226 = event-data() -> ("NewVal"=w353:bool)  [unwired: 1 in]
        n227 = case shown="False" w353 {
          tunnel: w352 -> [w362 _]
          tunnel: [w355 w373] -> w351
          tunnel: w350 -> [w354 w373]
          frame False {
            w369 = "Camera"
            w372 = FALSE ("Visible")
            n228 = local read "Camera Settings"() -> (w361:T2)
            n229 = Index Array(array=w362) -> (element=w365:cluster{string[]})  [unwired: 1 in]
            n230 = Unbundle(w361) -> ("Frame Rate"=w360:i32, "Compression"=w359:i32, "Size"=w363:u16)
            n231 = Unbundle(w365) -> (w364:string[])
            n232 = Index Array(array=w364, index=w363) -> (element=w358:string)
            n233 = call-poly <vilib>:"Write Key.vi"("section"=w369, "value"=w358, "key"="Size", "refnum"=w354) -> ("refnum out"=w371:T21)  [unwired: 2 in, 5 out]
            n234 = call-poly <vilib>:"Write Key.vi"("section"=w369, "value"=w360, "key"="FrameRate", "refnum"=w371) -> ("refnum out"=w370:T21)  [unwired: 1 in, 6 out]
            n235 = property on="Camera Settings" class="Clust (strict)"("Visible"=w372) -> ()  [unwired: 2 in, 2 out]
            n236 = local write "DB Camera Config"(w372) -> ()
            n237 = call-poly <vilib>:"Write Key.vi"("section"=w369, "value"=w359, "key"="Compression", "refnum"=w370) -> ("refnum out"=w356:T21)  [unwired: 1 in, 6 out]
            n238 = call <vilib>:"Close Config Data.vi"("refnum"=w356) -> ("file path"=w357:path)  [unwired: 2 in, 8 out]
            n239 = call <vilib>:"Open Config Data.vi"("configuration file path"=w357) -> ("refnum"=w355:T21)  [unwired: 8 in, 2 out]
          }
          frame True {
            n240 = property on="Camera Settings" class="Clust (strict)"("Visible"=TRUE) -> ()  [unwired: 2 in, 2 out]
          }
        }
      }
      event "Camera Settings": Value Change {
        # "Update summary string when any elements of DB camera change"
        n241 = event-data() -> ("NewVal"=w386:T2)  [unwired: 1 in]
        n242 = Index Array(array=w382) -> (element=w381:cluster{string[]})  [unwired: 1 in]
        n243 = Unbundle(w386) -> ("Frame Rate"=w377:i32, "Compression"=w376:i32, "Size"=w379:u16)
        n244 = Unbundle(w381) -> (w380:string[])
        n245 = Index Array(array=w380, index=w379) -> (element=w378:string)
        n246 = Format Into String(format string="%s   %dfps   %d%%", w378, w377, w376) -> (resulting string=w383:string)  [unwired: 2 in, 1 out]
        n247 = Build Array(w383) -> (w384:string[])
        n248 = property on="DB Camera Config" class="Bool (strict)"("Strings [4]"=w384) -> ()  [unwired: 2 in, 2 out]
      }
      event "Motor.Enable": Value Change {
        # "When the test mode otor enable helper is set, update that\ntree row item's value"
        n249 = event-data() -> ("NewVal"=w392:bool)  [unwired: 1 in]
        n250 = Unbundle("Motor") -> ("Value"=w391:dbl)  [unwired: 1 out]
        n251 = Select(t=w391, s=w392, f=0.0) -> (s? t:f=w389:dbl)
        n252 = call <vilib>:"NT Write Number.vi"("Numeric"=w389, "Name"=w388) -> ()  [unwired: 9 in, 1 out]
      }
      event "Test Slider": Value Change {
        # "When the test mode slider helper is set, update that\ntree row item's value"
        n253 = event-data() -> ("NewVal"=w395:dbl)  [unwired: 1 in]
        n254 = call <vilib>:"NT Write Number.vi"("Numeric"=w395, "Name"=w396) -> ()  [unwired: 9 in, 1 out]
      }
      event "On/Off": Value Change {
        # "When the test mode on/off helper value is set, update that\ntree row item's value"
        n255 = event-data() -> ("NewVal"=w400:bool)  [unwired: 1 in]
        n256 = Boolean To (0,1)(Boolean=w400) -> (0, 1=w399:i16)
        n257 = call <vilib>:"NT Write Number.vi"("Numeric"=w399, "Name"=w398) -> ()  [unwired: 9 in, 1 out]
      }
      event "Rev/Fwd": Value Change {
        # "When the test mode helper value for relays is set, update that\ntree row item's value"
        n258 = event-data() -> ("NewVal.Forward"=w408:bool, "NewVal.Reverse"=w407:bool)  [unwired: 1 in]
        n259 = Boolean To (0,1)(Boolean=w408) -> (0, 1=w404:i16)
        n260 = Boolean To (0,1)(Boolean=w407) -> (0, 1=w406:i16)
        n261 = Negate(x=w406) -> (-x=w405:i16)
        n262 = Add(x=w404, y=w405) -> (x+y=w403:i16)
        n263 = call <vilib>:"NT Write Number.vi"("Numeric"=w403, "Name"=w402) -> ()  [unwired: 9 in, 1 out]
      }
      event "Test Ring": Value Change {
        # "When a test mode helper value is selected from the ring,\nset the tree item's variable to the string value"
        n264 = event-data() -> ("NewVal"=w412:u16)  [unwired: 1 in]
        n265 = property on="Test Ring" class="Ring (strict)"() -> ("Strings []"=w413:string[])  [unwired: 2 in, 2 out]
        n266 = Index Array(array=w413, index=w412) -> (element=w411:string)
        n267 = call <vilib>:"NT Write String.vi"("String"=w411, "Name"=w410) -> ()  [unwired: 9 in, 1 out]
      }
      event "Rec Mode": Value Change {
        # "Update globals for recording mode and path to read log from.\nClear when logging and let NetworkTables set path for vision to\nuse."
        n268 = event-data() -> ("NewVal"=w423:enum32{"Stop", "Record", "Playback"})  [unwired: 1 in]
        n269 = global write "WPI_DashboardLogging Global.vi" "Logging Filename"(path "") -> ()
        n270 = case shown="\"Playback\"" w423 {
          tunnel: w422 -> [_ w425 w433]
          tunnel: [_ _ w432] -> w419
          tunnel: [_ _ w431] -> _
          tunnel: w417 -> [_ _ w429]
          tunnel: cluster{i32, i32} {-250, 170} -> [_ _ w428]
          tunnel: [_ _ T24 {"Image Size"=TRUE, "Image Type"=TRUE, "Pixel Value"=TRUE, "ROI Information"=TRUE, "Zoom Factor"=FALSE} ("Image Information Shown:All Elements")] -> w415
          tunnel: [_ _ TRUE ("Zoom Factor")] -> w414
          frame Default {
          }
          frame "Stop", "Record" {
            # "Place Window too"
            n271 = invoke class="VI" method="FP.Close"(reference=w425) -> (reference out=w424:refnum<vi>)  [unwired: 2 in, 2 out]
            n272 = invoke class="VI" method="Abort VI"(reference=w424) -> ()  [unwired: 2 in, 3 out]
          }
          frame "Playback" {
            n273 = call "Open Playback Panel.vi"("Offset"=w428, "DB VI Ref"=w429, "Playback in"=w433) -> ("Playback out"=w430:refnum<vi>)  [unwired: 8 in]
            n274 = register-events(w430) -> (reference out=w432:refnum<event-registration>, error out=w431:errorcluster)  [unwired: 2 in]
          }
        }
        n275 = global write "WPI_DashboardLogging Global.vi" "Recording"(w423) -> ()
        n276 = property on="Camera Image" class="ImageControl"("Image Information Shown"=w415, "Image Information Visible"=w414) -> ()  [unwired: 2 in, 2 out]
        n277 = call <vilib>:"WPI_DashboardNT Log FieldName Cache.vi"("Operation"=enum16{"Lookup/Add", "Index", "Clear"}."Clear") -> ()  [unwired: 8 in, 3 out]
      }
      event Panel Close {
        w434 = enum32{"Stop", "Record", "Playback"}."Stop" ("Rec Mode")
        # "Playback window has been closed, abort"
        n278 = event-data() -> ()  [unwired: 1 in, 4 out]
        n279 = local write "Rec Mode"(w434) -> ()
        n280 = global write "WPI_DashboardLogging Global.vi" "Recording"(w434) -> ()
      }
      event Panel Close {
        # "Abort playback window and ourself"
        n281 = event-data() -> ()  [unwired: 1 in, 4 out]
        n282 = invoke class="VI" method="FP.Close"(reference=w439) -> (reference out=w438:refnum<vi>)  [unwired: 2 in, 2 out]
        n283 = invoke class="VI" method="Abort VI"(reference=w438) -> (error out=w437:errorcluster)  [unwired: 2 in, 2 out]
        n284 = invoke class="VI" method="Abort VI"(error in=w437) -> ()  [unwired: 2 in, 3 out]
      }
      event "Vision": Value Change {
        # "Enable/Disable Compression slider.\nHW USB is hard-coded into the camera"
        n285 = event-data() -> ("NewVal"=w445:u16)  [unwired: 1 in]
        n286 = Equal?(x=w445, y=u32 2 ("milliseconds to wait")) -> (x = y?=w443:bool)
        n287 = Select(t=T25."Disabled and Grayed Out" ("Disabled"), s=w443, f=T25."Enabled" ("Disabled")) -> (s? t:f=w440:T25)
        n288 = property on="Compression" class="Slide (strict)"("DisabledEnum"=w440) -> ()  [unwired: 2 in, 2 out]
      }
    }
  }
  n289 = while {
    tunnel: w38 -> [w448]
    i -> [w451]
    stop <- FALSE stop-if-true
    n290 = Wait (ms)(milliseconds to wait=u32 100) -> ()  [unwired: 1 out]
    n291 = case shown="\"Playback\"" "Rec Mode" {
      tunnel: w451 -> [_ _ w466]
      tunnel: [u32 2829099 ("Base Color") u32 11141120 ("Target Color") w455] -> w447
      frame "Stop", Default {
        # "Reset the color, extra updates don't cost much"
      }
      frame "Record" {
      }
      frame "Playback" {
        # "Playback"
        n292 = Quotient & Remainder(x=w466, y=u32 50 ("milliseconds to wait")) -> (x-y*floor(x/y)=w462:u32)  [unwired: 1 out]
        n293 = Divide(x=w462, y=u32 50 ("milliseconds to wait")) -> (x/y=w459:dbl)
        n294 = Multiply(x=6.283185307179586, y=w459) -> (x*y=w464:dbl)
        n295 = Sine(x=w464) -> (sin(x)=w463:dbl)
        n296 = Absolute Value(x=w463) -> (abs(x)=w456:dbl)
        n297 = call "Interpolate RGB Color.vi"("Proportion"=w456, "Target Color"=u32 30976, "Base Color"=u32 2829099) -> ("Result Color"=w455:u32)  [unwired: 8 in]
      }
    }
    n298 = property class="Pane"(reference=w448, "PaneColor"=w447) -> ()  [unwired: 1 in, 2 out]
  }
  n299 = TCP Create Listener(10:u16 1741 ("timeout ms (25000)")) -> (3:w1:refnum<k5>)  [unwired: 4 in, 2 out]
  n300 = while {
    tunnel: w1 -> [w468]
    stop <- FALSE stop-if-true
    n301 = TCP Wait On Listener(11:w468) -> (4:w467:refnum<k5>)  [unwired: 3 in, 4 out]
    n302 = local write "TCP"(w467) -> ()
  }
  n303 = property on="On/Off" class="Bool (strict)"("Visible"=w6) -> ()  [unwired: 2 in, 2 out]
  n304 = property on="Motor" class="Clust (strict)"("Visible"=w6) -> ()  [unwired: 2 in, 2 out]
  n305 = property on="Progress" class="Clust (strict)"("Visible"=w6) -> ()  [unwired: 2 in, 2 out]
  n306 = property on="Test Ring" class="Ring (strict)"("Visible"=w6) -> ()  [unwired: 2 in, 2 out]
  n307 = property on="Rev/Fwd" class="Clust (strict)"("Visible"=w6) -> ()  [unwired: 2 in, 2 out]
  n308 = property on="Camera Settings" class="Clust (strict)"("Visible"=w6) -> ()  [unwired: 2 in, 2 out]
  n309 = local write "DB Camera Config"(w6) -> ()
  n310 = global write "WPI_DashboardLogging Global.vi" "Recording"(w32) -> ()
  n311 = local write "Rec Mode"(w32) -> ()
